vi "Reserve Device.vi"(0 "Session Handle in":T1, 11 "error in (no error)":errorcluster) -> (4 "Session Handle out":T1, 15 "error out":errorcluster)   [LabVIEW 2015, in "SLSC Switch.lvlib" / "SLSC Session.lvclass"]
uses:
  SLSC Session.lvclass
  Typedefs/Session Handle.ctl
  SLSC Session.lvclass/SLSC Session.ctl
  <vilib>/SLSC/SLSC.lvlib
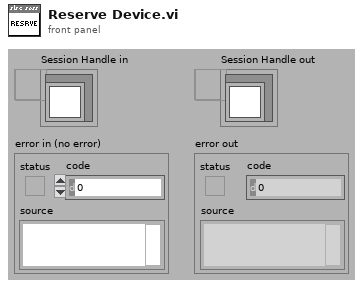
[diagram p1: front panel]
types:
  T1 = typedef "SLSC Switch.lvlib/SLSC Session.lvclass/Session Handle.ctl" = refnum<data-value>
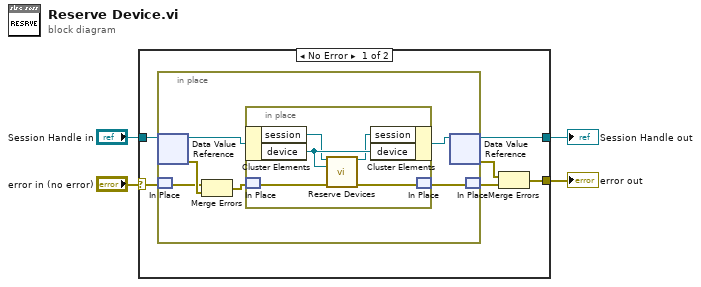
[diagram p0: block diagram]
diagram:
  n1 = case shown="No Error" "error in (no error)" {
    selector: "error in (no error)" -> [w5 w22]
    tunnel: "Session Handle in" -> [w10 w23]
    tunnel: [w9 w23] -> w3
    tunnel: [w6 w22] -> w2
    frame No Error {
      n2 = in-place {
        n3 = in-place-dvr #1(w10) -> (w14:refnum<class "SLSC Session.lvclass">, w16:errorcluster)
        n4 = in-place-match #2(w5) -> (w15:errorcluster)
        n5 = Merge Errors(w15, w16) -> (w12:errorcluster)
        n6 = in-place {
          n7 = in-place-cluster #3(w14) -> ("session"=w20:refnum<k21>, "device"=w21:refnum<k21>)
          n8 = in-place-match #4(w12) -> (w18:errorcluster)
          n9 = call <vilib>:"Reserve Devices.vi"("session in"=w20, "devices"=w21, "error in (no error)"=w18) -> ("session out"=w19:refnum<k21>, "error out"=w17:errorcluster)  [unwired: 11 in]
          n10 = in-place-cluster #3("session"=w19, "device"=w21) -> (w13:refnum<class "SLSC Session.lvclass">)
          n11 = in-place-match #4(w17) -> (w11:errorcluster)
        }
        n12 = in-place-dvr #1(w13) -> (w9:T1, w7:errorcluster)
        n13 = in-place-match #2(w11) -> (w8:errorcluster)
      }
      n14 = Merge Errors(w7, w8) -> (w6:errorcluster)
    }
    frame Error {
    }
  }
  "Session Handle out" <- w3
  "error out" <- w2
